vi "Run Execution Unit Count Checks.vi"(8 "error in":errorcluster, 9 "Test Configuration":T2, 10 "Target in":refnum<k24>, 11 "Create Execution Unit in":refnum<class "Create Execution Unit.lvclass">) -> (0 "error out":errorcluster, 3 "Create Execution Unit out":refnum<class "Create Execution Unit.lvclass">)   [LabVIEW 2020, in "Create Execution Unit.lvclass"]
uses:
  Create Execution Unit.lvclass
  Engine/Implementation/Execution Unit Factory/Execution Unit Factory.lvclass
  Shared/Data Word Format.ctl
  Engine/Custom Device/Logging Configuration.ctl
  Engine/Custom Device/Custom Device.lvlib
  Shared/Coupling Mode.ctl
  Shared/Bus Selection.ctl
  Shared/Initialization Method.ctl
  Shared/AIM Hardware Parameters.ctl
  Scripting/AIM MIL-STD-1553 Scripting.lvlib
  Engine/Implementation/Shared Resources/Shared Resources.lvclass
  Engine/Implementation/Shared Resources Factory/Shared Resources Factory.lvclass
  Shared/Address.ctl
  NationalInstruments.VeriStand.SystemDefinitionAPI
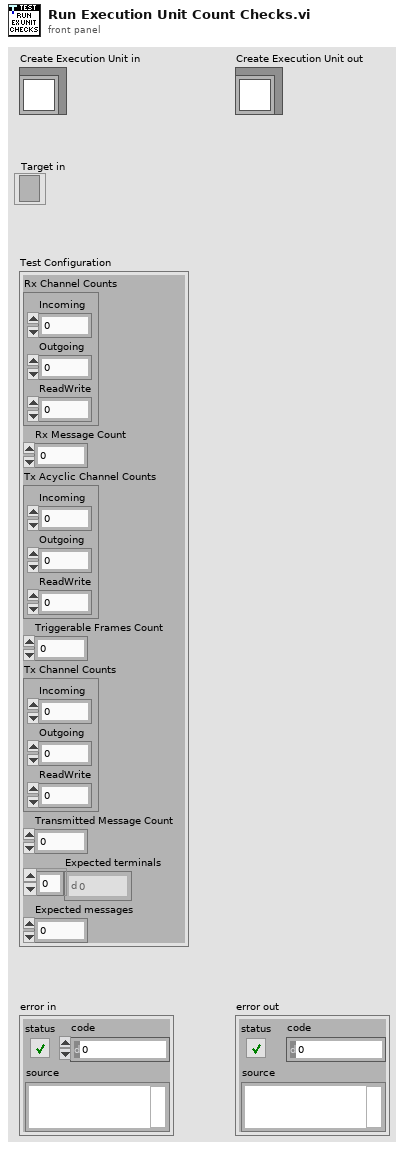
[diagram p1: front panel]
types:
  T1 = typedef "Address.ctl" = u16
  T2 = cluster{"Rx Channel Counts":cluster{"Incoming":i32, "Outgoing":i32, "ReadWrite":i32}, "Rx Message Count":i32, "Tx Acyclic Channel Counts":cluster{"Incoming":i32, "Outgoing":i32, "ReadWrite":i32}, "Triggerable Frames Count":i32, "Tx Channel Counts":cluster{"Incoming":i32, "Outgoing":i32, "ReadWrite":i32}, "Transmitted Message Count":i32, "Expected terminals":T1[], "Expected messages":i32}
  T3 = typedef "AIM Hardware Parameters.ctl" = cluster{"initialization method":T4, "card number":i32, "pxi slot number":i32, "biu number":i32, "bus selection":T5, "coupling mode":T6}
  T4 = typedef "Initialization Method.ctl" = enum16{"PXI Slot Number", "Card Number"}
  T5 = typedef "Bus Selection.ctl" = enum16{"Both", "Primary", "Secondary"}
  T6 = typedef "Coupling Mode.ctl" = enum16{"Isolated Onboard Termination", "Transformer Coupled", "Direct Coupled", "External with Onboard Termination", "Onboard Digital Wrap-around"}
  T7 = typedef "AIM MIL-STD-1553 Engine.lvlib/Custom Device.lvlib/Logging Configuration.ctl" = cluster{"configured":bool, "directory":string, "file name":string, "timestamp file name":bool, "data word format":T8}
  T8 = typedef "Data Word Format.ctl" = string
  T9 = cluster{"Incoming":i32, "Outgoing":i32, "ReadWrite":i32}
  T10 = typedef "Custom Device API.lvlib/Custom Device Item Ref.ctl" = u64
  T11 = typedef "AIM MIL-STD-1553 Engine.lvlib/Custom Device.lvlib/1553 Configuration.ctl" = cluster{"Bus Controller":T12, "Remote Terminals":T17[]}
  T12 = typedef "AIM MIL-STD-1553 Engine.lvlib/Custom Device.lvlib/Bus Controller Configuration.ctl" = cluster{"Simulated":bool, "Major Frames":map{u8, T13}, "Minor Frames":map{u8, T14}, "Acyclic Frames":map{u8, T15}, "Messages":map{u16, T16}}
  T13 = typedef "AIM MIL-STD-1553 Engine.lvlib/Custom Device.lvlib/Major Frame Configuration.ctl" = cluster{"Major Frame ID":u8, "Minor Frame IDs":u8[]}
  T14 = typedef "AIM MIL-STD-1553 Engine.lvlib/Custom Device.lvlib/Minor Frame Configuration.ctl" = cluster{"Minor Frame ID":u8, "Message IDs":u16[]}
  T15 = typedef "AIM MIL-STD-1553 Engine.lvlib/Custom Device.lvlib/Acyclic Frame Configuration.ctl" = cluster{"Acyclic Frame ID":u8, "Message IDs":u16[]}
  T16 = typedef "AIM MIL-STD-1553 Engine.lvlib/Custom Device.lvlib/Message Configuration.ctl" = cluster{"Transfer ID":u16, "Transfer Type":enum16{"BC to RT transfer", "RT to BC transfer", "RT to RT transfer"}, "Transmitting RT Address":u8, "Receiving RT Address":u8, "Transmitting RT Sub-address":u8, "Receiving RT Sub-address":u8, "Word Count / Mode Code":u8}
  T17 = typedef "AIM MIL-STD-1553 Engine.lvlib/Custom Device.lvlib/Remote Terminal Configuration.ctl" = cluster{"RT Address":u8, "Subaddress":cluster{"Value":u8, "Direction":T18, "Mode Code?":bool}[]}
  T18 = typedef "Direction.ctl" = enum16{"Rx", "Tx"}
  T19 = typedef "AIM MIL-STD-1553 Engine.lvlib/Interfaces.lvlib/Execution Unit Information.ctl" = cluster{"Execution Unit":refnum<class "Execution Unit.lvclass">, "Incoming Channels":T10[], "Outgoing Channels":T10[], "ReadWrite Channels":T10[]}
  T20 = cluster{"grouped asynchronous execution units":T19[]}[]
  T21 = cluster{"grouped asynchronous execution units":T19[]}
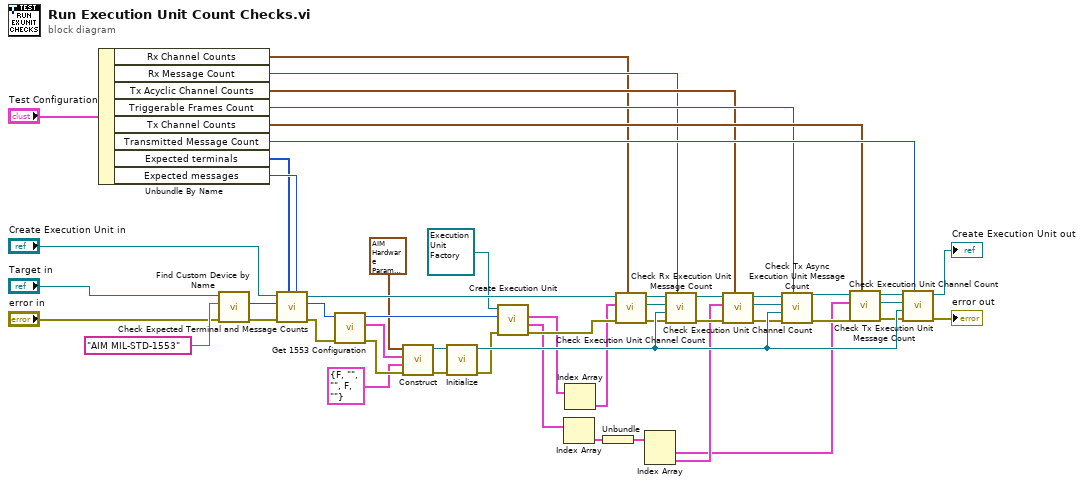
[diagram p0: block diagram]
diagram:
  n1 = Unbundle By Name("Test Configuration") -> ("Rx Channel Counts"=w46:T9, "Rx Message Count"=w47:i32, "Tx Acyclic Channel Counts"=w48:T9, "Triggerable Frames Count"=w49:i32, "Tx Channel Counts"=w50:T9, "Transmitted Message Count"=w51:i32, "Expected terminals"=w6:T1[], "Expected messages"=w7:i32)
  n2 = call "Find Custom Device by Name.vi"("error in"="error in", "custom device name"="AIM MIL-STD-1553" ("name"), "target"="Target in") -> ("error out"=w22:errorcluster, "custom device"=w21:T10)  [unwired: 5 in, 2 out]
  n3 = call "Check Expected Terminal and Message Counts.vi"("expected messages"=w7, "expected terminals"=w6, "error in"=w22, "custom device"=w21, "Create Execution Unit in"="Create Execution Unit in") -> ("error out"=w25:errorcluster, "custom device out"=w14:T10, "Create Execution Unit out"=w24:refnum<class "Create Execution Unit.lvclass">)  [unwired: 4 in]
  n4 = call "Get 1553 Configuration.vi"("error in"=w25, "custom device ref"=w14) -> ("error out"=w26:errorcluster, "1553 configuration out"=w15:T11, "custom device ref out"=w28:T10)  [unwired: 7 in]
  n5 = call "Construct.vi"("error in"=w26, "logging configuration"=T7 {"configured"=FALSE, "directory"="", "file name"="", "timestamp file name"=FALSE, "data word format"=""}, "1553 configuration"=w15, "hardware parameters"=T3 {"initialization method"=enum."PXI Slot Number", "card number"=0, "pxi slot number"=0, "biu number"=0, "bus selection"=enum."Both", "coupling mode"=enum."Isolated Onboard Termination"} ("device parameters")) -> ("error out"=w19:errorcluster, "shared resources out"=w20:refnum<class "Shared Resources.lvclass">)  [unwired: 6 in]
  n6 = call-dynamic "Initialize.vi"("error in"=w19, "shared resources"=w20) -> ("error out"=w27:errorcluster, "shared resources out"=w42:refnum<class "Shared Resources.lvclass">)  [unwired: 8 in]
  n7 = call-dynamic "Create Execution Unit.vi"("error in"=w27, "custom device ref"=w28, "execution unit factory"=refnum<class "Execution Unit Factory.lvclass"> refnum ("Execution Unit Factory Implementation in")) -> ("error out"=w44:errorcluster, "asynchronous execution units"=w5:T20, "inline execution units"=w11:T19[])  [unwired: 5 in, 1 out]
  n8 = Index Array(array=w5) -> (element=w4:T21)  [unwired: 1 in]
  n9 = Index Array(array=w11) -> (element=w23:T19)  [unwired: 1 in]
  n10 = Unbundle(w4) -> ("grouped asynchronous execution units"=w3:T19[])
  n11 = call "Check Execution Unit Channel Count.vi"("Channel Counts"=w46, "error in"=w44, "Execution Unit Information"=w23, "TestCase in"=w24) -> ("error out"=w31:errorcluster, "Execution Unit"=w29:refnum<class "Execution Unit.lvclass">, "TestCase out"=w30:refnum<class "Create Execution Unit.lvclass">)  [unwired: 5 in]
  n12 = Index Array(array=w3) -> (element #1=w1:T19, element #2=w2:T19)  [unwired: 2 in]
  n13 = call "Check Rx Execution Unit Message Count.vi"("Rx Message Count"=w47, "error in"=w31, "shared resources in"=w42, "Execution Unit"=w29, "Create Execution Unit in"=w30) -> ("error out"=w33:errorcluster, "Create Execution Unit out"=w32:refnum<class "Create Execution Unit.lvclass">)  [unwired: 4 in, 1 out]
  n14 = call "Check Execution Unit Channel Count.vi"("Channel Counts"=w48, "error in"=w33, "Execution Unit Information"=w2, "TestCase in"=w32) -> ("error out"=w34:errorcluster, "Execution Unit"=w35:refnum<class "Execution Unit.lvclass">, "TestCase out"=w36:refnum<class "Create Execution Unit.lvclass">)  [unwired: 5 in]
  n15 = call "Check Tx Async Execution Unit Message Count.vi"("Triggerable Frames Count"=w49, "error in"=w34, "shared resources in"=w42, "Execution Unit"=w35, "Create Execution Unit in"=w36) -> ("error out"=w38:errorcluster, "Create Execution Unit out"=w39:refnum<class "Create Execution Unit.lvclass">)  [unwired: 4 in, 1 out]
  n16 = call "Check Execution Unit Channel Count.vi"("Channel Counts"=w50, "error in"=w38, "Execution Unit Information"=w1, "TestCase in"=w39) -> ("error out"=w37:errorcluster, "Execution Unit"=w40:refnum<class "Execution Unit.lvclass">, "TestCase out"=w41:refnum<class "Create Execution Unit.lvclass">)  [unwired: 5 in]
  n17 = call "Check Tx Execution Unit Message Count.vi"("Transmitted Message Count"=w51, "error in"=w37, "shared resources in"=w42, "Execution Unit"=w40, "Create Execution Unit in"=w41) -> ("error out"=→"error out":errorcluster, "Create Execution Unit out"=→"Create Execution Unit out":refnum<class "Create Execution Unit.lvclass">)  [unwired: 4 in, 1 out]
